vi "ChangeComboBox(SubVI).vi"(8 "Error In":errorcluster, 9 "NumPlot":dbl, 10 "Name":string, 11 "Strings and Values In[]":cluster{"String":string, "Value":string}[](array[cluster])) -> (0 "Error Out":errorcluster, 3 "Strings and Values Out[]":cluster{"String":string, "Value":string}[](array[cluster]))   [LabVIEW 2018]
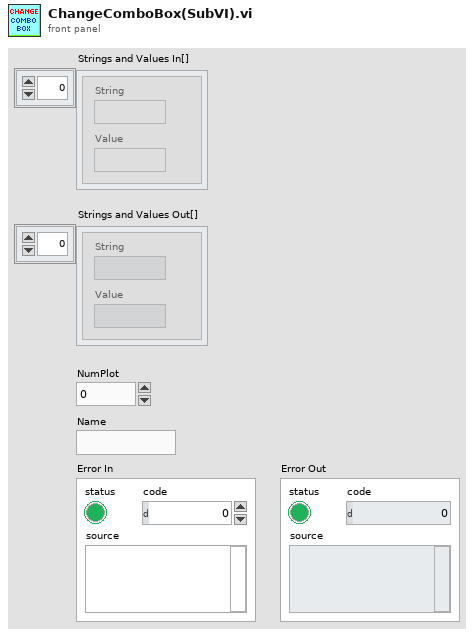
[diagram p1: front panel]
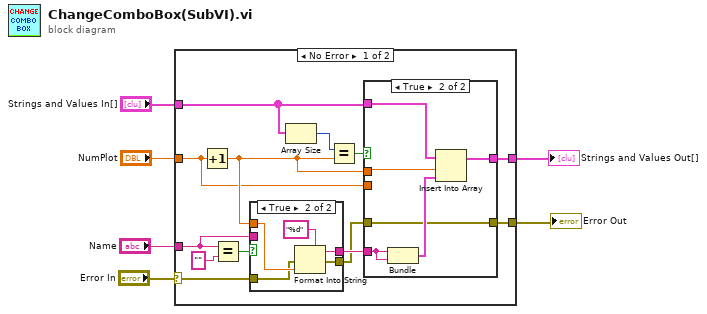
[diagram p0: block diagram]
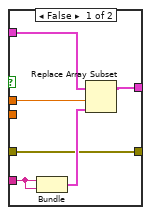
[diagram p2: hidden frame]
diagram:
  n1 = case shown="No Error" "Error In" {
    selector: "Error In" -> [w9 w39]
    tunnel: "Name" -> [w19 _]
    tunnel: [w15 _] -> w5
    tunnel: "NumPlot" -> [w12 _]
    tunnel: "Strings and Values In[]" -> [w10 _]
    tunnel: [w7 w39] -> w1
    frame No Error {
      n2 = Increment(x=w12) -> (x+1=w13:dbl)
      n3 = Equal?(x=w19, y="") -> (x = y?=w18:bool)
      n4 = case shown="True" w18 {
        tunnel: [w33 w37] -> w11
        tunnel: w19 -> [w33 _]
        tunnel: w13 -> [_ w36]
        tunnel: w9 -> [w32 w35]
        tunnel: [w32 w34] -> w8
        frame False {
        }
        frame True {
          n5 = Format Into String(format string="%d", error in=w35, w36) -> (resulting string=w37:string, error out=w34:errorcluster)  [unwired: 1 in]
        }
      }
      n6 = Array Size(array=w10) -> (size(s)=w16:i32)
      n7 = Equal?(x=w16, y=w13) -> (x = y?=w14:bool)
      n8 = case shown="True" w14 {
        tunnel: [w24 w30] -> w15
        tunnel: w10 -> [w23 w29]
        tunnel: w13 -> [w22 w28]
        tunnel: w12 -> [_ _]
        tunnel: w11 -> [w21 w27]
        tunnel: w8 -> [w20 w26]
        tunnel: [w20 w26] -> w7
        frame False {
          n9 = Bundle("Name"=w21, "Name"=w21) -> (w25:cluster{"Name":string, "Name":string})  [unwired: 1 in]
          n10 = Replace Array Subset(array=w23, new element=w25, index=w22) -> (w24:cluster{"String":string, "Value":string}[])
        }
        frame True {
          n11 = Bundle("Name"=w27, "Name"=w27) -> (w31:cluster{"Name":string, "Name":string})  [unwired: 1 in]
          n12 = Insert Into Array(array=w29, index=w28, new element=w31) -> (w30:cluster{"String":string, "Value":string}[])
        }
      }
    }
    frame Error {
    }
  }
  "Strings and Values Out[]" <- w5
  "Error Out" <- w1
